vi "Model Initial Values - Alternate Select Channels Dialog.vi"(4 "Selection Properties":T1, 6 "FP Win Title":string="Select Channels", 7 "Channel Label":string="System Channels", 8 "error in (no error)":errorcluster, 9 "Custom Filter":refnum<k24>, 10 "Filter":u8(ring)=1 items=["K_CHAN_R", "K_CHAN_W", "K_CHAN_RW", "K_CHAN_VOLT", "K_CHAN_FAULT", "K_ALL", "K_CUSTOM"], 11 "Start Item Ref":T2=18446744073709551615 format="%.0x") -> (0 "error out":errorcluster, 1 "Canceled":bool, 2 "Channel Names":string[](array[string]), 3 "Channel Paths":string[](array[string]))   [LabVIEW 2011, in "Model Initial Values Custom Device.lvlib"]
uses:
  Model Initial Values Custom Device.lvlib
  <vilib>/NI Veristand/Custom Device API/Custom Device Item Ref.ctl
  NationalInstruments.VeriStand.SystemStorageUI
  NationalInstruments.VeriStand.SystemStorage
  <vilib>/NI Veristand/Custom Device API/Custom Device API.lvlib
panel:
  in  "OK":bool
  in  "Cancel":bool
  in  "System Channels":refnum<k24>(container)
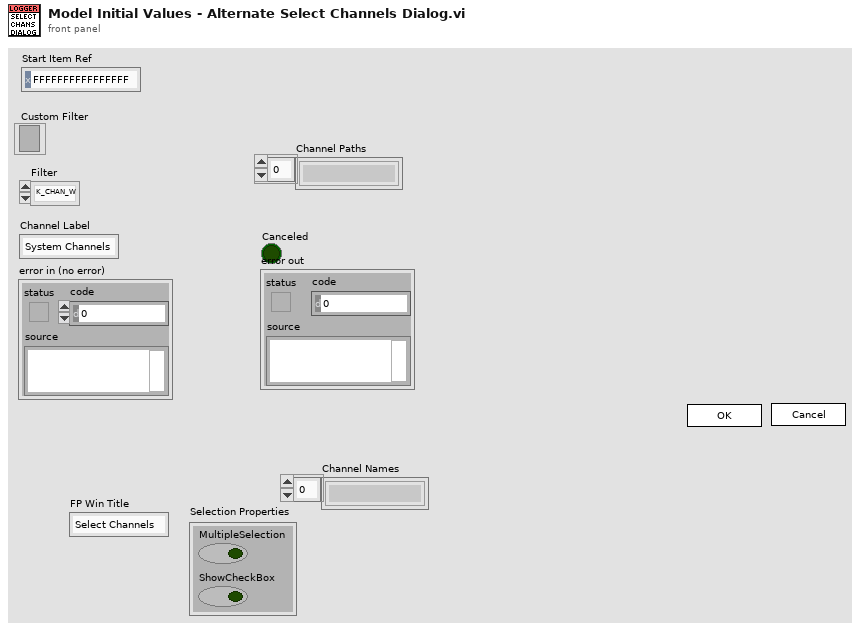
[diagram p1: front panel]
types:
  T1 = cluster{"MultipleSelection":bool, "ShowCheckBox":bool}
  T2 = typedef "Custom Device API.lvlib/Custom Device Item Ref.ctl" = u64
  T3 = cluster{"Shut Down":bool, "Error":errorcluster, "Root":refnum<k24>, "Cancel":bool, "MapTree":cluster{"Ref":refnum<k24>, "Filter":refnum<k24>}, "Channel Paths":string[], "Channel Names":string[]}
  T4 = typedef "Custom Device API.lvlib/Custom Device Pointer.ctl" = refnum<k24>
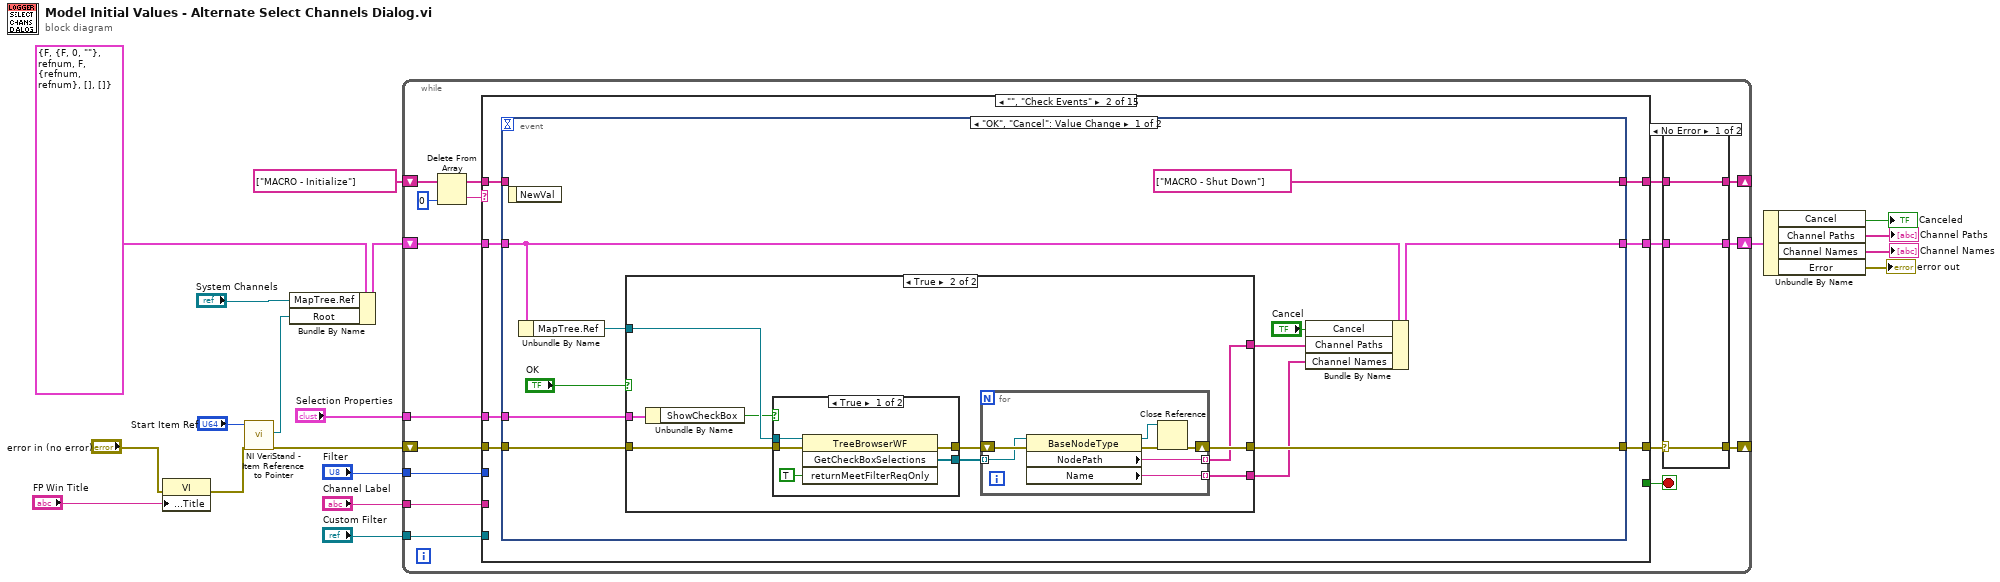
[diagram p0: block diagram]
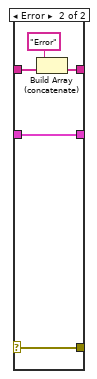
[diagram p2: hidden frame]
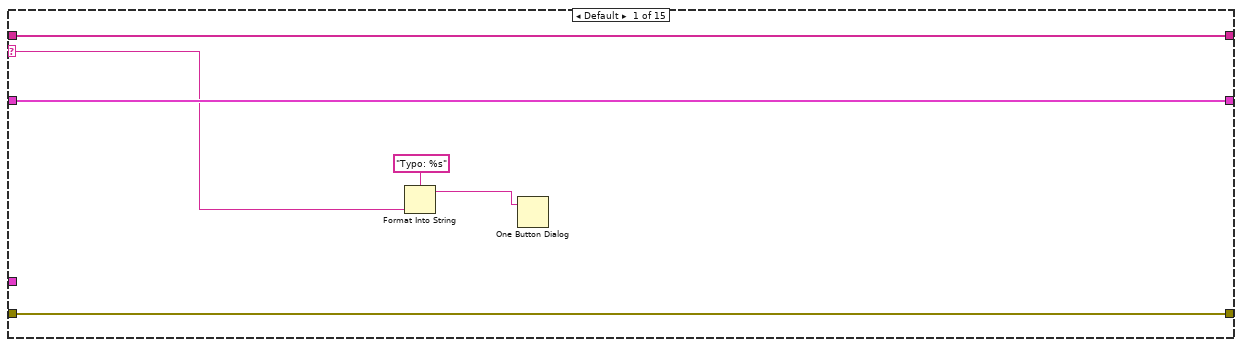
[diagram p3: hidden frame]
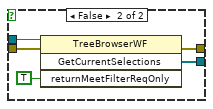
[diagram p5: hidden frame]
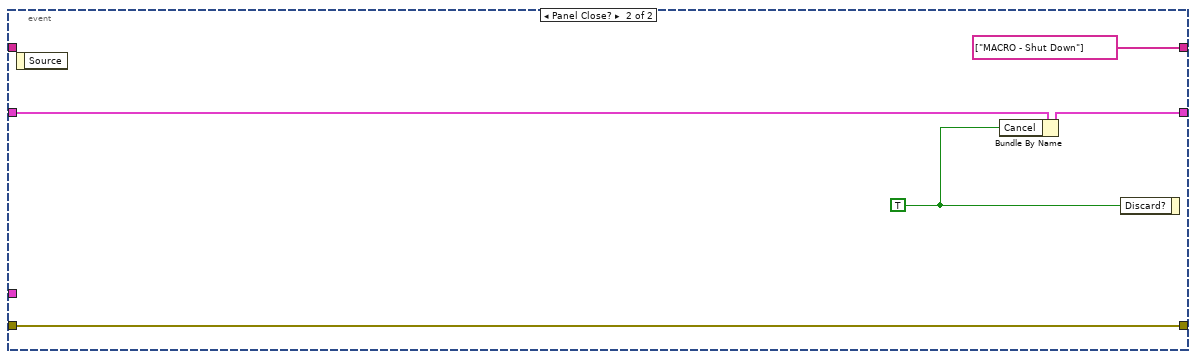
[diagram p6: hidden frame]
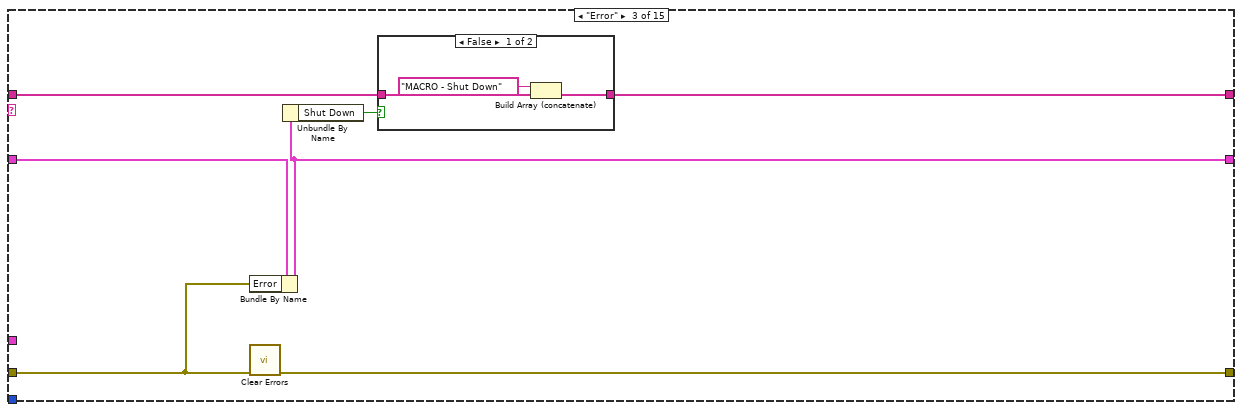
[diagram p7: hidden frame]
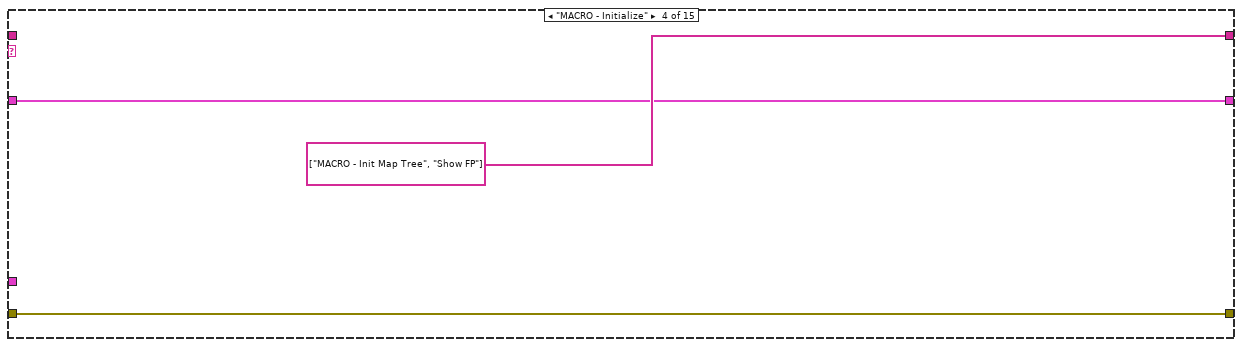
[diagram p9: hidden frame]
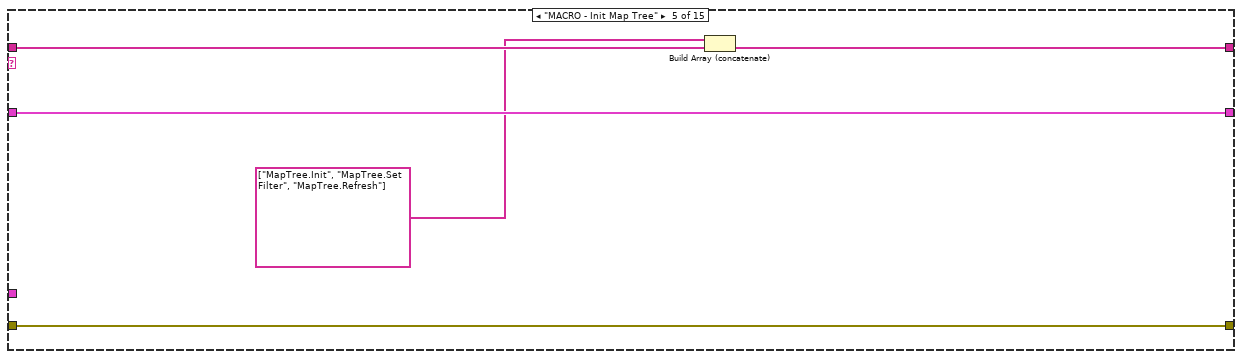
[diagram p10: hidden frame]
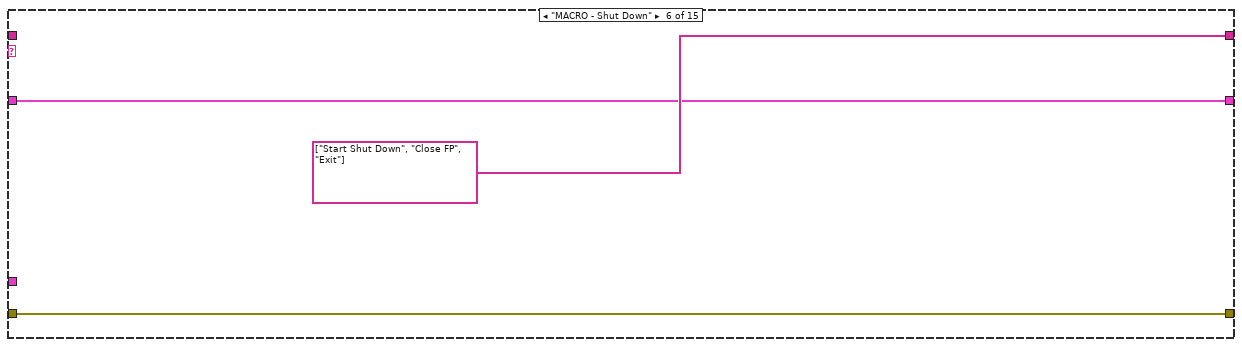
[diagram p11: hidden frame]
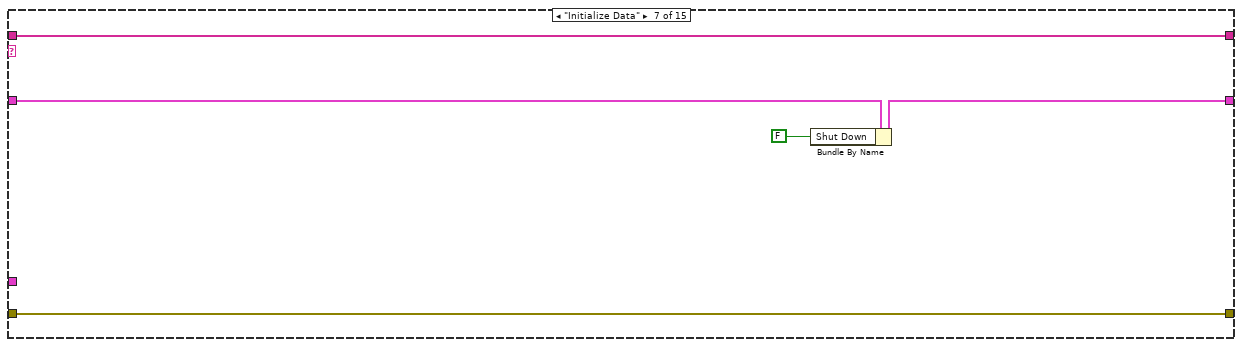
[diagram p12: hidden frame]
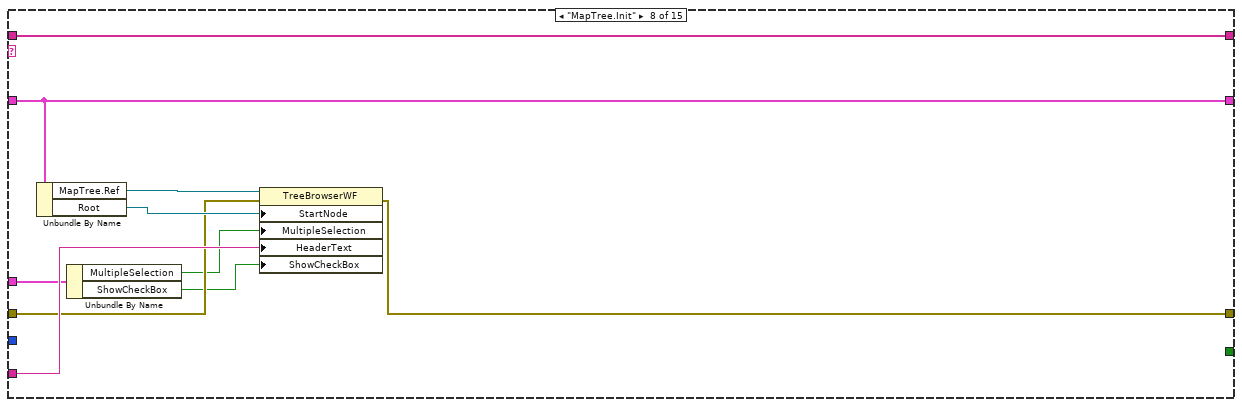
[diagram p13: hidden frame]
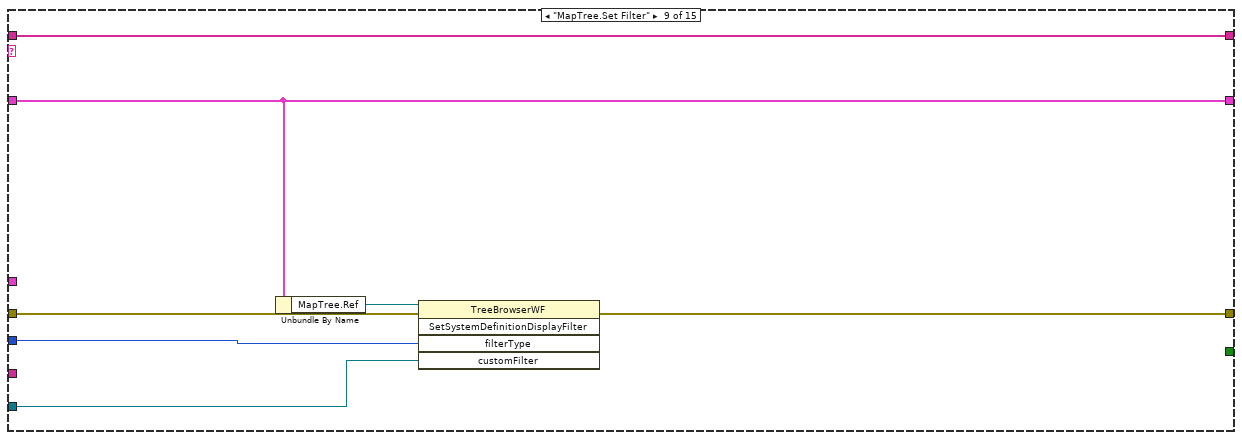
[diagram p14: hidden frame]
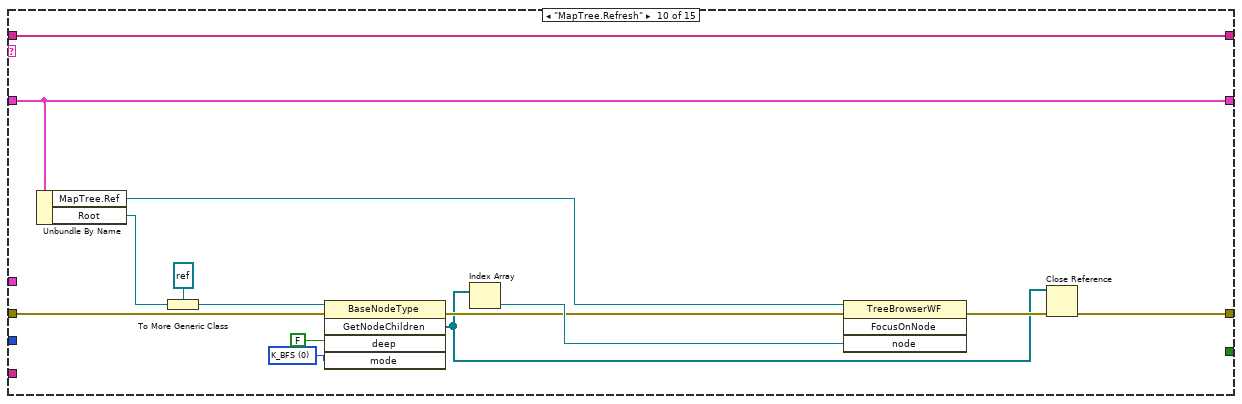
[diagram p15: hidden frame]
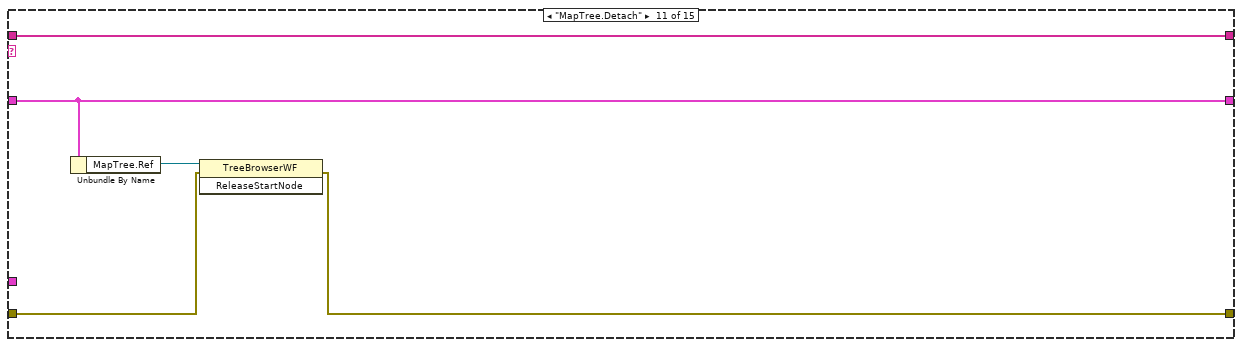
[diagram p16: hidden frame]
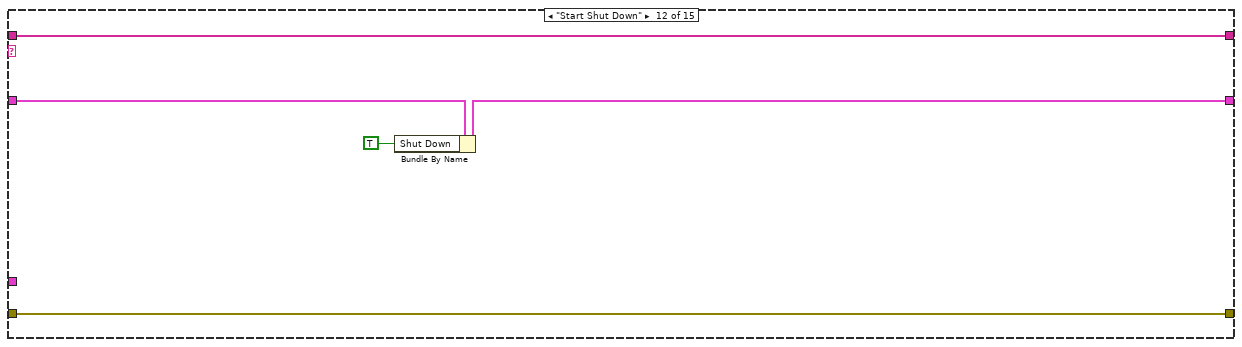
[diagram p17: hidden frame]
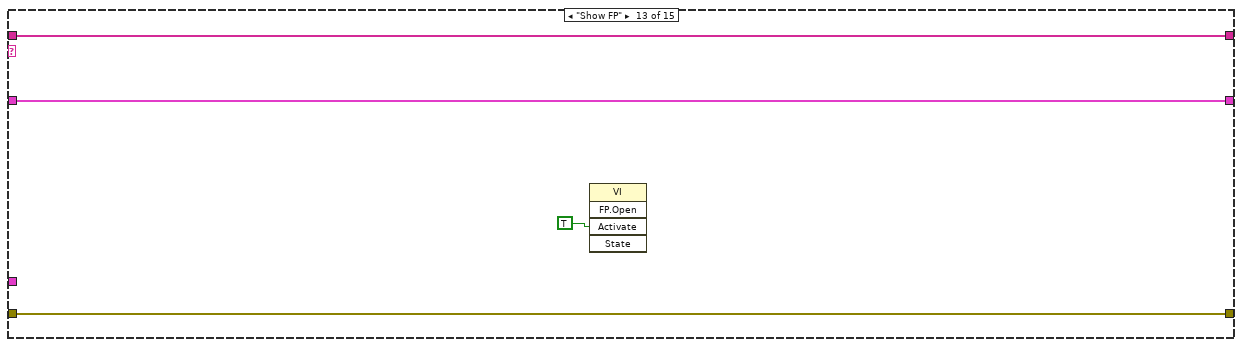
[diagram p18: hidden frame]
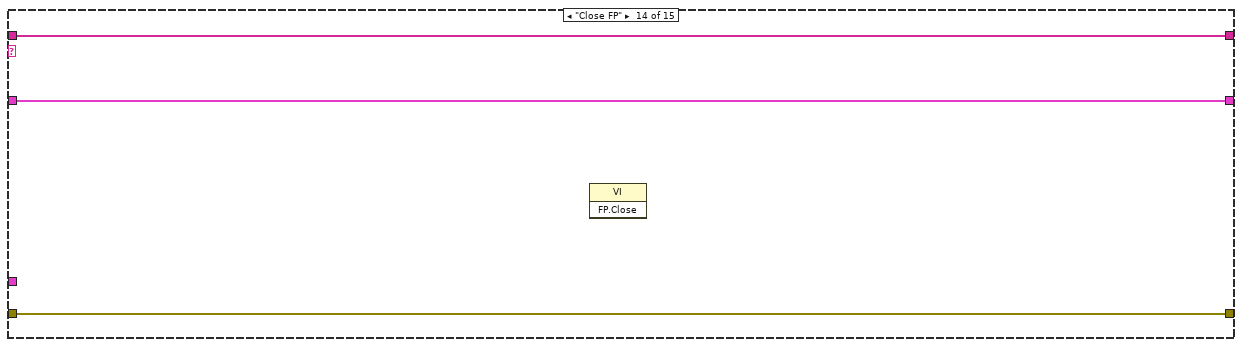
[diagram p19: hidden frame]
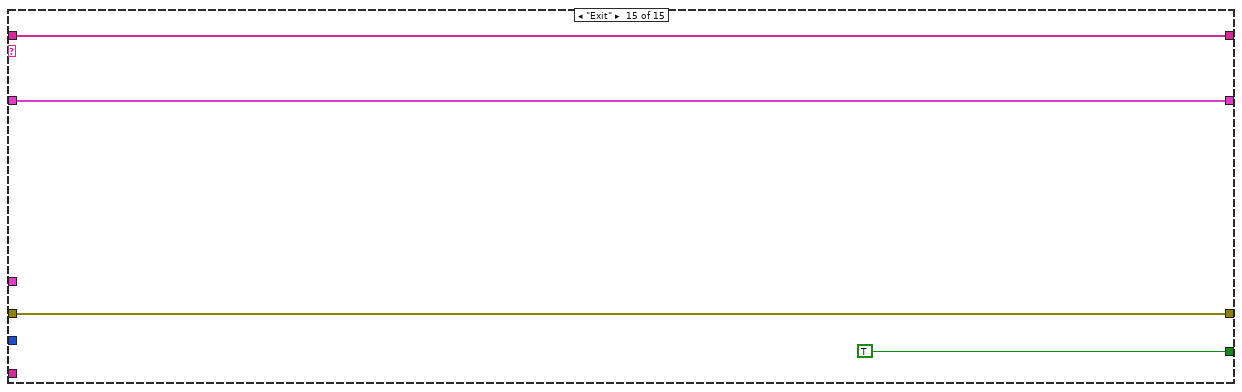
[diagram p20: hidden frame]
diagram:
  n1 = property class="VI"(error in="error in (no error)", "Front Panel.Title"="FP Win Title") -> (error out=w6:errorcluster)  [unwired: 1 in, 1 out]
  n2 = call <vilib>:"NI VeriStand - Item Reference to Pointer.vi"("error in (no error)"=w6, "Item Ref in"="Start Item Ref") -> ("error out"=w9:errorcluster, "Node Pointer"=w8:T4)  [unwired: 6 in, 2 out]
  n3 = Bundle By Name(cluster=T3 {"Shut Down"=FALSE, "Error"={"status"=FALSE, "code"=0, "source"=""}, "Root"=refnum, "Cancel"=FALSE, "MapTree"={"Ref"=refnum, "Filter"=refnum}, "Channel Paths"=[], "Channel Names"=[]} ("State Data"), "MapTree.Ref"="System Channels", "Root"=w8) -> (w16:T3)
  n4 = while {
    shift-right: [w26] -> _
    shift-left: string[] ["MACRO - Initialize"] -> [w36]
    shift-right: [w28] -> _
    shift-left: w9 -> [w32]
    shift-right: [w25] -> w13
    shift-left: w16 -> [w30]
    tunnel: "Channel Label" -> [w23]
    tunnel: "Filter" -> [w22]
    tunnel: "Custom Filter" -> [w21]
    tunnel: "Selection Properties" -> [w20]
    stop <- w31 stop-if-true
    n5 = Delete From Array(array=w36, index=0) -> (deleted portion=w33:string, array with subset deleted=w34:string[])  [unwired: 1 in]
    n6 = case shown="\"\", \"Check Events\"" w33 {
      selector: w33 -> [w46 _ _ _ _ _ _ _ _ _ _ _ _ _ _]
      tunnel: w34 -> [w50 w57 w104 _ w119 _ w127 w137 w144 w158 w163 w164 w172 w175 w179]
      tunnel: [w50 w52 w103 string[] ["MACRO - Init Map Tree", "Show FP"] ("array") w116 string[] ["Start Shut Down", "Close FP", "Exit"] ("array") w127 w137 w144 w158 w163 w164 w172 w175 w179] -> w27
      tunnel: [w49 w55 w101 w114 w118 w122 w126 w131 w142 w150 w159 w168 w171 w174 w178] -> w29
      tunnel: w32 -> [w49 w54 w102 w114 w118 w122 w126 w132 w140 w156 w160 w168 w171 w174 w178]
      tunnel: [_ _ _ _ _ _ _ _ _ _ _ _ _ _ TRUE] -> w31
      tunnel: w30 -> [w48 w56 w107 w112 w117 w120 w123 w136 w141 w157 w162 w167 w170 w173 w176]
      tunnel: [w48 w53 w106 w112 w117 w120 w125 w136 w141 w157 w162 w166 w170 w173 w176] -> w24
      tunnel: w23 -> [_ _ _ _ _ _ _ w133 _ _ _ _ _ _ _]
      tunnel: w22 -> [_ _ _ _ _ _ _ _ w139 _ _ _ _ _ _]
      tunnel: w21 -> [_ _ _ _ _ _ _ _ w138 _ _ _ _ _ _]
      tunnel: w20 -> [_ w51 _ _ _ _ _ w130 _ _ _ _ _ _ _]
      frame Default {
        n7 = Format Into String(format string="Typo: %s", w46) -> (resulting string=w45:string)  [unwired: 2 in, 1 out]
        n8 = One Button Dialog(message=w45) -> ()  [unwired: 1 in, 1 out]
      }
      frame "", "Check Events" {
        n9 = event shown="[0] \"OK\", \"Cancel\": Value Change" {
          selector: _ -> [_ _]
          dyn-events: _ -> [_ _]
          timeout: _ -> [_ _]
          tunnel: [w62 w100] -> w55
          tunnel: w54 -> [w64 w100]
          tunnel: [w67 w97] -> w53
          tunnel: w56 -> [w65 w99]
          tunnel: w57 -> [_ _]
          tunnel: [string[] ["MACRO - Shut Down"] string[] ["MACRO - Shut Down"]] -> w52
          tunnel: w51 -> [w59 _]
          event "OK", "Cancel": Value Change {
            n10 = event-data() -> ()  [unwired: 1 in, 1 out]
            n11 = Unbundle By Name(w65) -> ("MapTree.Ref"=w60:refnum<k24>)
            n12 = case shown="True" "OK" {
              tunnel: w60 -> [_ w78]
              tunnel: w64 -> [w69 w77]
              tunnel: [_ w73] -> w63
              tunnel: [w69 w74] -> w62
              tunnel: w59 -> [_ w72]
              tunnel: [_ w70] -> w58
              frame False {
              }
              frame True {
                n13 = Unbundle By Name(w72) -> ("ShowCheckBox"=w71:bool)
                n14 = case shown="True" w71 {
                  tunnel: w78 -> [w83 w88]
                  tunnel: w77 -> [w82 w87]
                  tunnel: [w80 w85] -> w76
                  tunnel: [w79 w84] -> w75
                  frame True {
                    n15 = invoke class="TreeBrowserWF" method="GetCheckBoxSelections"(reference=w83, error in=w82, "returnMeetFilterReqOnly"=TRUE) -> (error out=w80:errorcluster, "GetCheckBoxSelections"=w79:refnum<k24>[])  [unwired: 1 in, 2 out]
                  }
                  frame False {
                    n16 = invoke class="TreeBrowserWF" method="GetCurrentSelections"(reference=w88, error in=w87, "returnMeetFilterReqOnly"=TRUE) -> (error out=w85:errorcluster, "GetCurrentSelections"=w84:refnum<k24>[])  [unwired: 1 in, 2 out]
                  }
                }
                n17 = for {
                  shift-right: [w90] -> w74
                  shift-left: w76 -> [w95]
                  tunnel: w75 -> [w94] mode=indexing
                  tunnel: [w93] -> w73 mode=indexing
                  tunnel: [w89] -> w70 mode=indexing
                  n18 = property class="BaseNodeType"(reference=w94, error in=w95) -> (reference out=w91:refnum<k24>, error out=w92:errorcluster, "NodePath"=w93:string, "Name"=w89:string)
                  n19 = Close Reference(reference=w91, error in (no error)=w92) -> (error out=w90:errorcluster)
                }
              }
            }
            n20 = Bundle By Name(cluster=w65, "Cancel"="Cancel", "Channel Paths"=w63, "Channel Names"=w58) -> (w67:T3)
          }
          event Panel Close? {
            w96 = TRUE ("Discard?")
            n21 = event-data() -> ()  [unwired: 1 in, 1 out]
            n22 = Bundle By Name(cluster=w99, "Cancel"=w96) -> (w97:T3)
            n23 = event-data("Discard?"=w96) -> ()  [unwired: 1 in, 1 out]
          }
        }
      }
      frame "Error" {
        n24 = Bundle By Name(cluster=w107, "Error"=w102) -> (w106:T3)
        n25 = call <vilib>:"Clear Errors.vi"("error in (no error)"=w102) -> ("error out"=w101:errorcluster)  [unwired: 6 in]
        n26 = Unbundle By Name(w106) -> ("Shut Down"=w105:bool)
        n27 = case shown="False" w105 {
          tunnel: w104 -> [w109 w111]
          tunnel: [w108 w111] -> w103
          frame False {
            n28 = Build Array (concatenate)("MACRO - Shut Down", w109) -> (w108:string[])
          }
          frame True {
            # "Do not interrupt a shut down sequence. This can cause an infinite loop."
          }
        }
      }
      frame "MACRO - Initialize" {
      }
      frame "MACRO - Init Map Tree" {
        n29 = Build Array (concatenate)(string[] ["MapTree.Init", "MapTree.Set Filter", "MapTree.Refresh"] ("array"), w119) -> (w116:string[])
      }
      frame "MACRO - Shut Down" {
      }
      frame "Initialize Data" {
        n30 = Bundle By Name(cluster=w123, "Shut Down"=FALSE) -> (w125:T3)
      }
      frame "MapTree.Init" {
        n31 = Unbundle By Name(w136) -> ("MapTree.Ref"=w135:refnum<k24>, "Root"=w134:refnum<k24>)
        n32 = Unbundle By Name(w130) -> ("MultipleSelection"=w129:bool, "ShowCheckBox"=w128:bool)
        n33 = property class="TreeBrowserWF"(reference=w135, error in=w132, "StartNode"=w134, "MultipleSelection"=w129, "HeaderText"=w133, "ShowCheckBox"=w128) -> (error out=w131:errorcluster)  [unwired: 1 out]
      }
      frame "MapTree.Set Filter" {
        n34 = Unbundle By Name(w141) -> ("MapTree.Ref"=w143:refnum<k24>)
        n35 = invoke class="TreeBrowserWF" method="SetSystemDefinitionDisplayFilter"(reference=w143, error in=w140, "filterType"=w139, "customFilter"=w138) -> (error out=w142:errorcluster)  [unwired: 1 in, 4 out]
      }
      frame "MapTree.Refresh" {
        w146 = 0 items=["K_BFS", "K_DFS", "K_CHILDONLY", "K_UP"] ("mode")
        n36 = Unbundle By Name(w157) -> ("MapTree.Ref"=w148:refnum<k24>, "Root"=w155:refnum<k24>)
        n37 = To More Generic Class(target class=refnum<k24> refnum, reference=w155) -> (generic class reference=w153:refnum<k24>)
        n38 = invoke class="BaseNodeType" method="GetNodeChildren"(reference=w153, error in=w156, "deep"=FALSE, "mode"=w146) -> (error out=w149:errorcluster, "GetNodeChildren"=w145:refnum<k24>[])  [unwired: 1 in, 3 out]
        n39 = Index Array(array=w145) -> (element=w152:refnum<k24>)  [unwired: 1 in]
        n40 = invoke class="TreeBrowserWF" method="FocusOnNode"(reference=w148, error in=w149, "node"=w152) -> (error out=w151:errorcluster)  [unwired: 1 in, 3 out]
        n41 = Close Reference(reference=w145, error in (no error)=w151) -> (error out=w150:errorcluster)
      }
      frame "MapTree.Detach" {
        n42 = Unbundle By Name(w162) -> ("MapTree.Ref"=w161:refnum<k24>)
        n43 = invoke class="TreeBrowserWF" method="ReleaseStartNode"(reference=w161, error in=w160) -> (error out=w159:errorcluster)  [unwired: 1 in, 2 out]
      }
      frame "Start Shut Down" {
        n44 = Bundle By Name(cluster=w167, "Shut Down"=TRUE) -> (w166:T3)
      }
      frame "Show FP" {
        n45 = invoke class="VI" method="FP.Open"("Activate"=TRUE ("Activate?")) -> ()  [unwired: 4 in, 5 out]
      }
      frame "Close FP" {
        n46 = invoke class="VI" method="FP.Close"() -> ()  [unwired: 3 in, 3 out]
      }
      frame "Exit" {
      }
    }
    n47 = case shown="No Error" w29 {
      selector: w29 -> [w39 w44]
      tunnel: [w39 w44] -> w28
      tunnel: w27 -> [w38 w42]
      tunnel: [w38 w41] -> w26
      tunnel: [w37 w43] -> w25
      tunnel: w24 -> [w37 w43]
      frame No Error {
      }
      frame Error {
        n48 = Build Array (concatenate)("Error", w42) -> (w41:string[])
      }
    }
  }
  n49 = Unbundle By Name(w13) -> ("Cancel"=→"Canceled":bool, "Channel Paths"=→"Channel Paths":string[], "Channel Names"=→"Channel Names":string[], "Error"=→"error out":errorcluster)
